vi "Vision Processing.vi"(4 "error in (no error)":errorcluster, 5 "Camera Type":enum16{"206", "1011"}(ring), 6 "Camera Name":string="Camera") -> ()   [LabVIEW 2012]
uses:
  Robot Global Data.vi
  <vilib>/vision/NI_Vision_Development_Module.lvlib
panel:
  in  "View":bool
  out "Target Info":T1(array[cluster])
  in  "Area Size Limit %":dbl=0.5
  in  "Particle Count Limit":i32=8
  in  "Score Limits":T2={"Rect Coverage"=60.0, "X Edge Strength"=40.0, "Y Edge Strength"=60.0, "Center"=32.0, "Outer"=50.0}
  in  "Processing":enum32{"Color", "Monochrome"}(tab)
  out "Value":cluster{i32, i32}
  out "Saturation":cluster{i32, i32}
  out "Hue":cluster{i32, i32}
  in  "Luminance":i32=10
  in  "Saturation":i32
  in  "Hue":i32(knob)=255 scale=0.0..255.0
  in  "Margins":cluster{"Hue":i32, "Sat":i32, "Val":i32}={"Hue"=26, "Sat"=9, "Val"=10} {"Sat" scale=0.0..80.0; "Val" scale=0.0..80.0; "Hue" scale=0.0..80.0}
  in  "Range":cluster{"Lower value":sgl, "Upper value":sgl}={"Lower value"=150.0, "Upper value"=255.0} {"Lower value" scale=0.0..255.0; "Upper value" scale=0.0..255.0}
  in  "View":bool
  out "Processed Image":T3(plugin-control)
  out "Original Image":T3(plugin-control)
  # "Instructions:\nProcessing the reflective tape that is illuminated by a ring light can be based\non color or light intensity.\nParticles within the image are scored by rectangle coverage, aspect ratio, and\nfor being hollow with a bold edge. A particle is considered a target if all scores\nare above the score limits. Particles can be annotated -- surrounded by\na rectangle and scores drawn to the left .\nTo control the number of particles being scored, use the count limit and the size\nlimit."
  # "To debug, Enable using the View button.\nFor color processing, you can click in the image to select the color for processing."
  # "Enable by clicking the View button.\nGreen scores are above the limit, orange are below. Inner/outer rect\nindicates all passed."
  # "Lower/Upper"
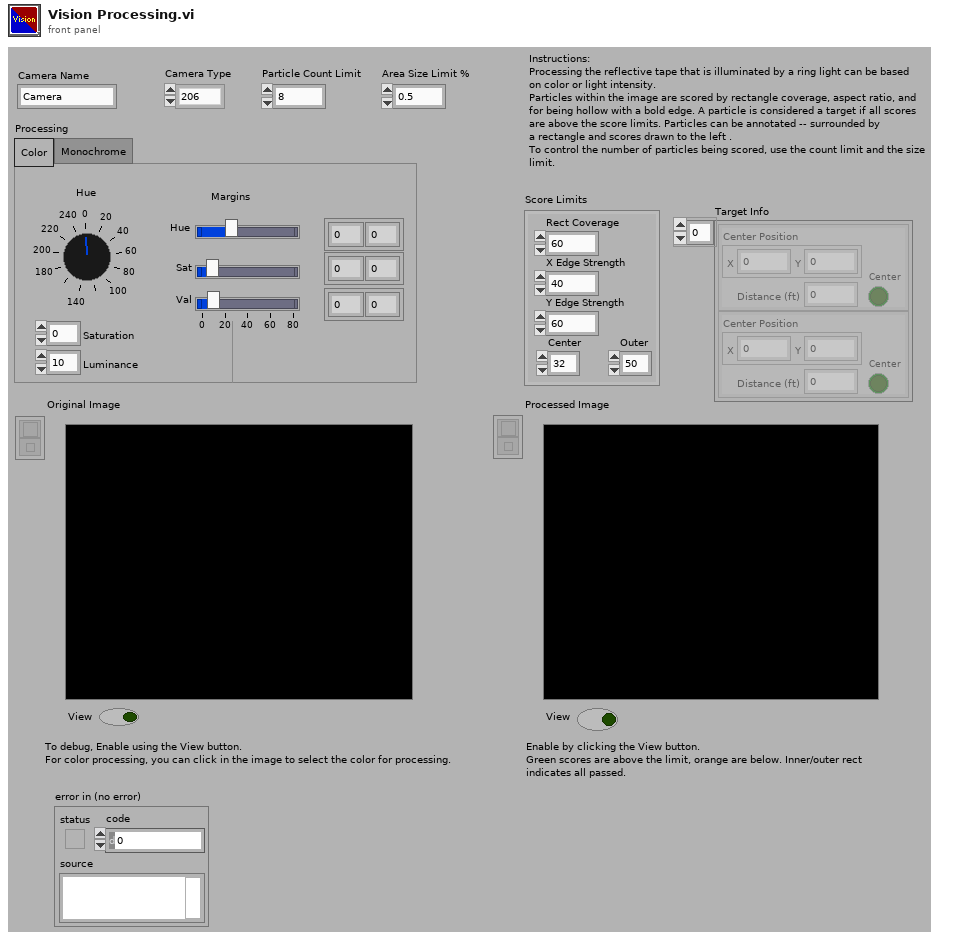
[diagram p1: front panel]
types:
  T1 = cluster{"Center Position":cluster{"X":dbl, "Y":dbl}, "Distance (ft)":dbl, "Center":bool}[]
  T2 = cluster{"Rect Coverage":dbl, "X Edge Strength":dbl, "Y Edge Strength":dbl, "Center":dbl, "Outer":dbl}
  T3 = typedef "IMAQ Image.ctl" = refnum<image>
  T4 = typedef "Image Type" = u32
  T5 = typedef "WPI_CameraDevRef.ctl" = cluster{"Camera Address":string, "CameraStatus":errorcluster, "Acquire Image Notifier":refnum<notifier>}
  T6 = cluster{"Position":cluster{"X":dbl, "Y":dbl}, "Distance (ft)":dbl, "Center":bool}[]
  T7 = typedef "WPI_CameraImageSize.ctl" = enum16{"640x480", "320x240", "160x120"}
  T8 = cluster{cluster{"Left":dbl, "Top":dbl, "Right":dbl, "Bottom":dbl}, "Scores":dbl[], cluster{"Long":dbl, "Short":dbl}}[]
  T9 = cluster{"Target Center (-1 to 1)":cluster{"X":dbl, "Y":dbl}, "Distance (ft)":dbl, "Center Target":bool}
  T10 = cluster{"Target Center (-1 to 1)":cluster{"X":dbl, "Y":dbl}, "Distance (ft)":dbl, "Center Target":bool}[]
  T11 = cluster{"Left":dbl, "Top":dbl, "Right":dbl, "Bottom":dbl}
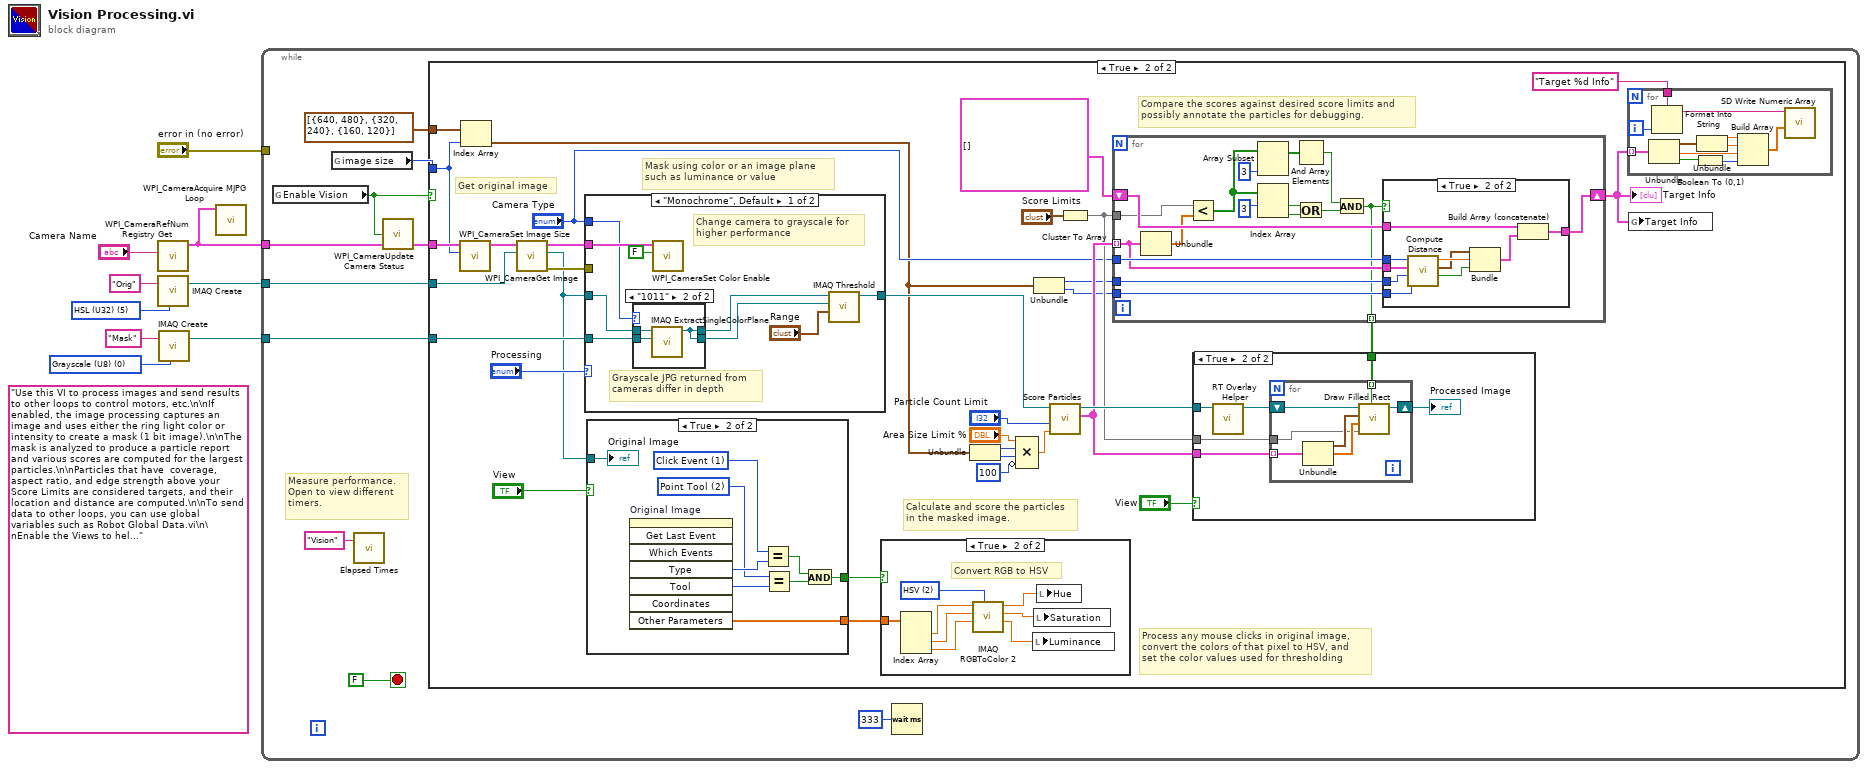
[diagram p0: block diagram]
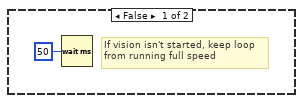
[diagram p2: hidden frame]
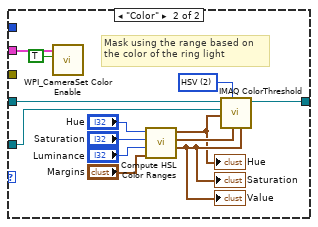
[diagram p5: hidden frame]
diagram:
  w3 = T4 0 items=["Grayscale (U8)", "Grayscale (I16)", "Grayscale (SGL)", "Complex (CSG)", "RGB (U32)", "HSL (U32)", "RGB (U64)", "Grayscale (U16)"] ("Image Type")
  (unwired) "Use this VI to process images and send results to other loops to control motors, etc.\n\nIf enabled, the image processing captures an image and uses either the ring light color or intensity to create a mask (1 bit image).\n\nThe mask is analyzed to produce a particle report and various scores are computed for the largest particles.\n\nParticles that have  coverage, aspect ratio, and edge strength above your Score Limits are considered targets, and their location and distance are computed.\n\nTo send data to other loops, you can use global variables such as Robot Global Data.vi\n\nEnable the Views to help debug color settings. Disable the View to speed up processing."
  w8 = T4 5 items=["Grayscale (U8)", "Grayscale (I16)", "Grayscale (SGL)", "Complex (CSG)", "RGB (U32)", "HSL (U32)", "RGB (U64)", "Grayscale (U16)"] ("Image Type")
  n1 = call <vilib>:"WPI_CameraRefNum Registry Get.vi"("refnum name"="Camera Name") -> ("CameraDevRef"=w5:T5)  [unwired: 9 in, 1 out]
  n2 = call "IMAQ Create"("Image Name"="Orig", "Image Type"=w8) -> ("New Image"=w7:T3)  [unwired: 2 in, 2 out]
  n3 = call "IMAQ Create"("Image Name"="Mask", "Image Type"=w3) -> ("New Image"=w1:T3)  [unwired: 2 in, 2 out]
  n4 = call <vilib>:"WPI_CameraAcquire MJPG Loop.vi"("CameraDevRef"=w5) -> ()  [unwired: 11 in]
  n5 = while {
    tunnel: w7 -> [w18]
    tunnel: w5 -> [w17]
    tunnel: "error in (no error)" -> [_]
    tunnel: w1 -> [w12]
    stop <- FALSE stop-if-true
    # "Measure performance.\nOpen to view different\ntimers."
    n6 = global read "Robot Global Data.vi" "Enable Vision"() -> (w15:bool)
    n7 = global read "Robot Global Data.vi" "image size"() -> (w13:T7)
    n8 = call "Elapsed Times.vi"("Call Name"="Vision") -> ()  [unwired: 2 in, 1 out]
    n9 = call <vilib>:"WPI_CameraUpdate Camera Status.vi"("CameraDevRef In"=w17, "Enable Vision"=w15) -> ("CameraDevRef Out"=w16:T5)  [unwired: 3 in]
    n10 = case shown="True" w15 {
      tunnel: w18 -> [_ w46]
      tunnel: w16 -> [_ w42]
      tunnel: w13 -> [_ w37]
      tunnel: w12 -> [_ w33]
      tunnel: cluster{i32, i32}[] [{640, 480}, {320, 240}, {160, 120}] -> [_ w36]
      frame False {
        # "If vision isn't started, keep loop\nfrom running full speed"
        n11 = Wait (ms)(milliseconds to wait=u32 50) -> ()  [unwired: 1 out]
      }
      frame True {
        # "Compare the scores against desired score limits and\npossibly annotate the particles for debugging."
        # "Process any mouse clicks in original image,\nconvert the colors of that pixel to HSV, and\nset the color values used for thresholding"
        # "Calculate and score the particles\nin the masked image."
        # "Mask using color or an image plane\nsuch as luminance or value"
        # "Get original image"
        n12 = call <vilib>:"WPI_CameraSet Image Size.vi"("Image Size"=w37, "CameraDevRef"=w42) -> ("CameraDevRef Out"=w43:T5)  [unwired: 8 in, 1 out]
        n13 = Index Array(array=w36, index=w37) -> (element=w21:cluster{i32, i32})
        n14 = call <vilib>:"WPI_CameraGet Image.vi"("Image"=w46, "CameraDevRef"=w43) -> ("error out"=w44:errorcluster, "Image Out"=w32:T3, "CameraDevRef Out"=w45:T5)  [unwired: 7 in]
        n15 = case shown="\"Monochrome\", Default" "Processing" {
          tunnel: w32 -> [w77 w99]
          tunnel: [w80 w98] -> w40
          tunnel: w45 -> [w78 w91]
          tunnel: w44 -> [_ _]
          tunnel: w33 -> [w76 w89]
          tunnel: "Camera Type" -> [w75 _]
          frame "Monochrome", Default {
            # "Grayscale JPG returned from\ncameras differ in depth"
            # "Change camera to grayscale for\nhigher performance"
            n16 = case shown="\"1011\"" w75 {
              tunnel: w77 -> [w83 w86]
              tunnel: w76 -> [w82 w85]
              tunnel: [w83 w84] -> w74
              tunnel: [w82 w84] -> w73
              frame "206", Default {
              }
              frame "1011" {
                n17 = call "IMAQ ExtractSingleColorPlane"("Image Dst"=w85, "Image Src"=w86) -> ("Image Dst Out"=w84:T3)  [unwired: 8 in, 1 out]
              }
            }
            n18 = call <vilib>:"WPI_CameraSet Color Enable.vi"("Color Enabled"=FALSE, "CameraDevRef"=w78) -> ()  [unwired: 8 in, 2 out]
            n19 = call "IMAQ Threshold"("Range"="Range", "Image Dst"=w73, "Image Src"=w74) -> ("Image Dst Out"=w80:T3)  [unwired: 3 in, 5 out]
          }
          frame "Color" {
            w97 = u16 2 items=["RGB", "HSL", "HSV", "HSI"] ("Color Mode")
            # "Mask using the range based on\nthe color of the ring light"
            n20 = call <vilib>:"WPI_CameraSet Color Enable.vi"("Color Enabled"=TRUE, "CameraDevRef"=w91) -> ()  [unwired: 8 in, 2 out]
            n21 = call "Compute HSL Color Ranges.vi"("Margins"="Margins", "Luminance"="Luminance", "Saturation"="Saturation", "Hue"="Hue") -> ("Lum Range"=w88:cluster{i32, i32}, "Sat Range"=w96:cluster{i32, i32}, "Hue Range"=w87:cluster{i32, i32})  [unwired: 5 in]
            "Hue" <- w87
            "Saturation" <- w88
            "Value" <- w88
            n22 = call "IMAQ ColorThreshold"("Blue or Luma or Val or Inten Range"=w88, "Green or Sat Range"=w96, "Color Mode"=w97, "Red or Hue Range"=w87, "Image Dst"=w89, "Image Src"=w99) -> ("Image Dst Out"=w98:T3)  [unwired: 4 in, 1 out]
          }
        }
        n23 = case shown="True" "View" {
          tunnel: w32 -> [_ w121]
          tunnel: [_ w116] -> w39
          tunnel: [_ w113] -> w38
          frame False {
          }
          frame True {
            w114 = 2 items=["None", "Selection Tool", "Point Tool", "Line Tool", "Rectangle Tool", "Oval Tool", "Polygon Tool", "ClosedFreehandTool", "Annulus Tool", "Rotated Rectangle Tool", "Zoom Tool", "Pan Tool", "Polyline Tool", "Freehand Tool"] ("Tool")
            w115 = 1 items=["No Event"=0, "Click Event"=1, "Draw Event"=2, "Size Event"=4, "Scroll Event"=5, "Double Click Event"=8] ("Type")
            n24 = invoke on="Original Image" class="ImageControl" method="Get Last Event"() -> ("Type"=w117:i32, "Tool"=w120:i32, "Other Parameters"=w113:sgl[])  [unwired: 8 in, 5 out]
            n25 = Equal?(x=w115, y=w117) -> (x = y?=w118:bool)
            n26 = Equal?(x=w114, y=w120) -> (x = y?=w119:bool)
            n27 = And(x=w118, y=w119) -> (x .and. y?=w116:bool)
            "Original Image" <- w121
          }
        }
        n28 = case shown="True" w39 {
          tunnel: w38 -> [_ w72]
          frame False {
          }
          frame True {
            w71 = u16 2 items=["RGB", "HSL", "HSV", "HSI", "CIE L*a*b*", "CIE XYZ"] ("Color Mode")
            # "Convert RGB to HSV"
            n29 = Index Array(array=w72) -> (element #1=w70:sgl, element #2=w68:sgl, element #3=w66:sgl)  [unwired: 3 in]
            n30 = call "IMAQ RGBToColor 2"("Color Mode"=w71, "Blue value"=w66, "Green value"=w68, "Red value"=w70) -> ("Blue or Luma or Val or Inten or Z or b*value"=w65:dbl, "Green or Sat or Y or a* value"=w67:dbl, "Red or Hue or X or L* value"=w69:dbl)  [unwired: 4 in, 1 out]
            n31 = local write "Luminance"(w65) -> ()
            n32 = local write "Saturation"(w67) -> ()
            n33 = local write "Hue"(w69) -> ()
          }
        }
        n34 = Unbundle(w21) -> (w25:i32, w24:i32)
        n35 = Compound Arithmetic op=MULTIPLY("Area Size Limit %", w25, w24, invert 100 ("length")) -> (w22:dbl)
        n36 = Unbundle(w21) -> (w35:i32, w34:i32)
        n37 = call "Score Particles.vi"("Area Size Limit"=w22, "Particle Count Limit"="Particle Count Limit", "Image Refnum in"=w40) -> ("Scored Particle Info"=w50:T8, "Image Refnum out"=w52:T3)  [unwired: 7 in]
        n38 = Cluster To Array(cluster="Score Limits") -> (array=w48:dbl[])
        n39 = for {
          shift-right: [w137] -> w29
          shift-left: T6 [] -> [w138]
          tunnel: w35 -> [w136]
          tunnel: w50 -> [w131] mode=indexing
          tunnel: w48 -> [w133]
          tunnel: "Camera Type" -> [w135]
          tunnel: w34 -> [w132]
          tunnel: [w122] -> w27 mode=indexing
          n40 = Unbundle(w131) -> ("Scores"=w134:dbl[])  [unwired: 2 out]
          n41 = Less?(x=w133, y=w134) -> (x < y?=w123:bool[])
          n42 = Array Subset(array=w123, length=3) -> (w125:bool[])  [unwired: 1 in]
          n43 = Index Array(array=w123, index #1=3 ("length")) -> (element #1=w127:bool, element #2=w128:bool)  [unwired: 1 in]
          n44 = And Array Elements(Boolean array=w125) -> (logical AND=w130:bool)
          n45 = Or(x=w127, y=w128) -> (x .or. y?=w129:bool)
          n46 = And(x=w130, y=w129) -> (x .and. y?=w122:bool)
          n47 = case shown="True" w122 {
            tunnel: w138 -> [w139 w149]
            tunnel: [w139 w148] -> w137
            tunnel: w136 -> [_ w146]
            tunnel: w135 -> [_ w144]
            tunnel: w132 -> [_ w143]
            tunnel: w131 -> [_ w141]
            frame False {
            }
            frame True {
              n48 = call "Compute Distance.vi"("Y Image Resolution"=w143, "X Image Resolution"=w146, "Particle Scores"=w141, "Camera Type"=w144) -> ("Center Target"=w140:bool, "Target Center (-1 to 1)"=w142:cluster{"X":dbl, "Y":dbl}, "Distance (ft)"=w145:dbl)  [unwired: 5 in]
              n49 = Bundle("Target Center (-1 to 1)"=w142, "Distance (ft)"=w145, "Center Target"=w140) -> (w147:T9)  [unwired: 1 in]
              n50 = Build Array (concatenate)(w149, w147) -> (w148:T10)
            }
          }
        }
        "Target Info" <- w29
        n51 = case shown="True" "View" {
          tunnel: w52 -> [_ w102]
          tunnel: w50 -> [_ w104]
          tunnel: w48 -> [_ w103]
          tunnel: w27 -> [_ w100]
          frame False {
          }
          frame True {
            n52 = call "RT Overlay Helper.vi"("Refnum in"=w102) -> ("Refnum out"=w105:T3)  [unwired: 10 in]
            n53 = for {
              shift-right: [w111] -> w101
              shift-left: w105 -> [w112]
              tunnel: w104 -> [w108] mode=indexing
              tunnel: w103 -> [w107]
              tunnel: w100 -> [w106] mode=indexing
              n54 = Unbundle(w108) -> (w109:T11, "Scores"=w110:dbl[])  [unwired: 1 out]
              n55 = call "Draw Filled Rect.vi"("Limit Passed"=w106, "Limits"=w107, "Scores"=w110, "Bounding Box"=w109, "image in"=w112) -> ("image out"=w111:T3)  [unwired: 6 in]
            }
            "Processed Image" <- w101
          }
        }
        n56 = for {
          tunnel: w29 -> [w64] mode=indexing
          tunnel: "Target %d Info" ("Name") -> [w63]
          i -> [w60]
          n57 = Unbundle(w64) -> ("Position"=w61:cluster{"X":dbl, "Y":dbl}, "Distance (ft)"=w56:dbl, "Center"=w59:bool)
          n58 = Format Into String(format string=w63, w60) -> (resulting string=w62:string)  [unwired: 2 in, 1 out]
          n59 = Boolean To (0,1)(Boolean=w59) -> (0, 1=w55:i16)
          n60 = Unbundle(w61) -> ("X"=w58:dbl, "Y"=w57:dbl)
          n61 = Build Array(w58, w57, w56, w55) -> (w54:dbl[])
          n62 = call <vilib>:"SD Write Numeric Array.vi"("Numeric Array"=w54, "Name"=w62) -> ()  [unwired: 8 in, 2 out]
        }
        n63 = global write "Robot Global Data.vi" "Target Info"(w29) -> ()
      }
    }
    n64 = Wait (ms)(milliseconds to wait=u32 333) -> ()  [unwired: 1 out]
  }
